vi "Numeric Limit Compare Runtime Test.vi"() -> (0 "error out":errorcluster, 2 "Pass":bool)   [LabVIEW 2015, in "Numeric Limit Compare Tests.lvlib"]
uses:
  Numeric Limit Compare Tests.lvlib
  Config/Comparison Types.ctl
  Config/Numeric Limit Compare Config.lvclass
  <vilib>/NI/Tag Bus/tag/Data Type.ctl
  <vilib>/NI/Tag Bus Module Framework/channel/channel classification.ctl
  classes/Step/Execution/StepState.ctl
  classes/Step/Execution/Step State Enum.ctl
  classes/Step/Execution/Step Flow Control.ctl
  Config/Numeric Limit Compare Config.lvclass/Numeric Limit Compare Config.ctl
  <vilib>/NI/Tag Bus/tag/tag descriptor.lvclass/tag descriptor.ctl
  <vilib>/NI/Tag Bus/table/data polymorphs/write one/write Double.vi
  <vilib>/NI/Tag Bus/table/data polymorphs/read one/read Boolean.vi
  Config/Write channel.vi
  Config/Write Comparison Type.vi
  Config/Write Lower Limit.vi
  Config/Write Negate Result.vi
  Config/Write Upper Limit_Limit.vi
  Config/Write Result Channel.vi
  <vilib>/NI/Tag Bus/tag/read tag name.vi
  <vilib>/NI/Tag Bus/tag/read data type.vi
  <vilib>/NI/Tag Bus/dictionary/locate tag.vi
  classes/Step/Execution/Step.lvclass
  <vilib>/NI/Tag Bus Module Framework/channel/TBM channel.lvclass
  <vilib>/NI/Tag Bus/tag/tag descriptor.lvclass
  <vilib>/NI/Tag Bus/dictionary/data dictionary.lvclass
  <vilib>/NI/Tag Bus/table/data table.lvlib
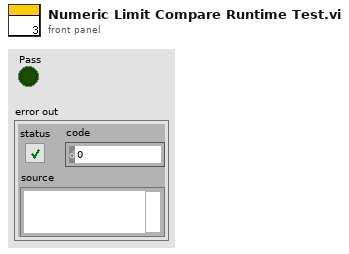
[diagram p1: front panel]
types:
  T1 = typedef "Comparison Types.ctl" = enum16{"GELE (>=<=)", "GTLE(><=)", "GTLT(><)", "GELT(>=<)", "EQ(==)", "NE (!=)", "GT(>)", "LT(<)", "GE(>=)", "LE(<=)"}
  T2 = typedef "Step.lvclass/StepState.ctl" = cluster{"Step State":T3, "Flow Control":T4, "Jump Index":i32}
  T3 = typedef "Step.lvclass/Step State Enum.ctl" = enum16{"Start", "Skipped", "Timeout", "Completed", "Running", "Aborted"}
  T4 = typedef "Step.lvclass/Step Flow Control.ctl" = enum16{"Next Step", "Jump"}
  T5 = typedef "TBM channel.lvclass/channel classification.ctl" = enum16{"input data", "output data", "processing parameter", "processing result"}
  T6 = typedef "tag bus.lvlib/tag descriptor.lvclass/Data Type.ctl" = enum16{"Double", "Single", "I64", "I32", "I16", "I8", "U64", "U32", "U16", "U8", "Boolean", "String", "Array of Double", "Array of Single", "Array of I64", "Array of I32", "Array of I16", "Array of I8", "Array of U64", "Array of U32", "Array of U16", "Array of U8", "Array of Boolean", "Array of String"}
  T7 = typedef "TBM channel.lvclass/data tables.ctl" = cluster{"input data":T8, "processing parameter":T8, "processing result":T8, "output data":T8}
  T8 = typedef "tag bus.lvlib/dictionary table pair.ctl" = cluster{"data dictionary":refnum<class "data dictionary.lvclass">, "data table":T9}
  T9 = typedef "tag bus.lvlib/data table.lvlib/data table.ctl" = cluster{"Double":dbl[], "Single":sgl[], "I64":i64[], "I32":i32[], "I16":i16[], "I8":i8[], "U64":u64[], "U32":u32[], "U16":u16[], "U8":u8[], "Boolean":bool[], "String":string[], "Array of Double":cluster{"DBL Array":dbl[]}[], "Array of Single":cluster{"SGL Array":sgl[]}[], "Array of I64":cluster{"I64 Array":i64[]}[], "Array of I32":cluster{"I32 Array":i32[]}[], "Array of I16":cluster{"I16 Array":i16[]}[], "Array of I8":cluster{"I8 Array":i8[]}[], "Array of U64":cluster{"U64 Array":u64[]}[], "Array of U32":cluster{"U32 Array":u32[]}[], "Array of U16":cluster{"U16 Array":u16[]}[], "Array of U8":cluster{"U8 Array":u8[]}[], "Array of Boolean":cluster{"Boolean Array":bool[]}[], "Array of String":cluster{"String Array":string[]}[]}
  T10 = cluster{"Step State":bool, "Flow Control":bool, "Jump Index":bool}
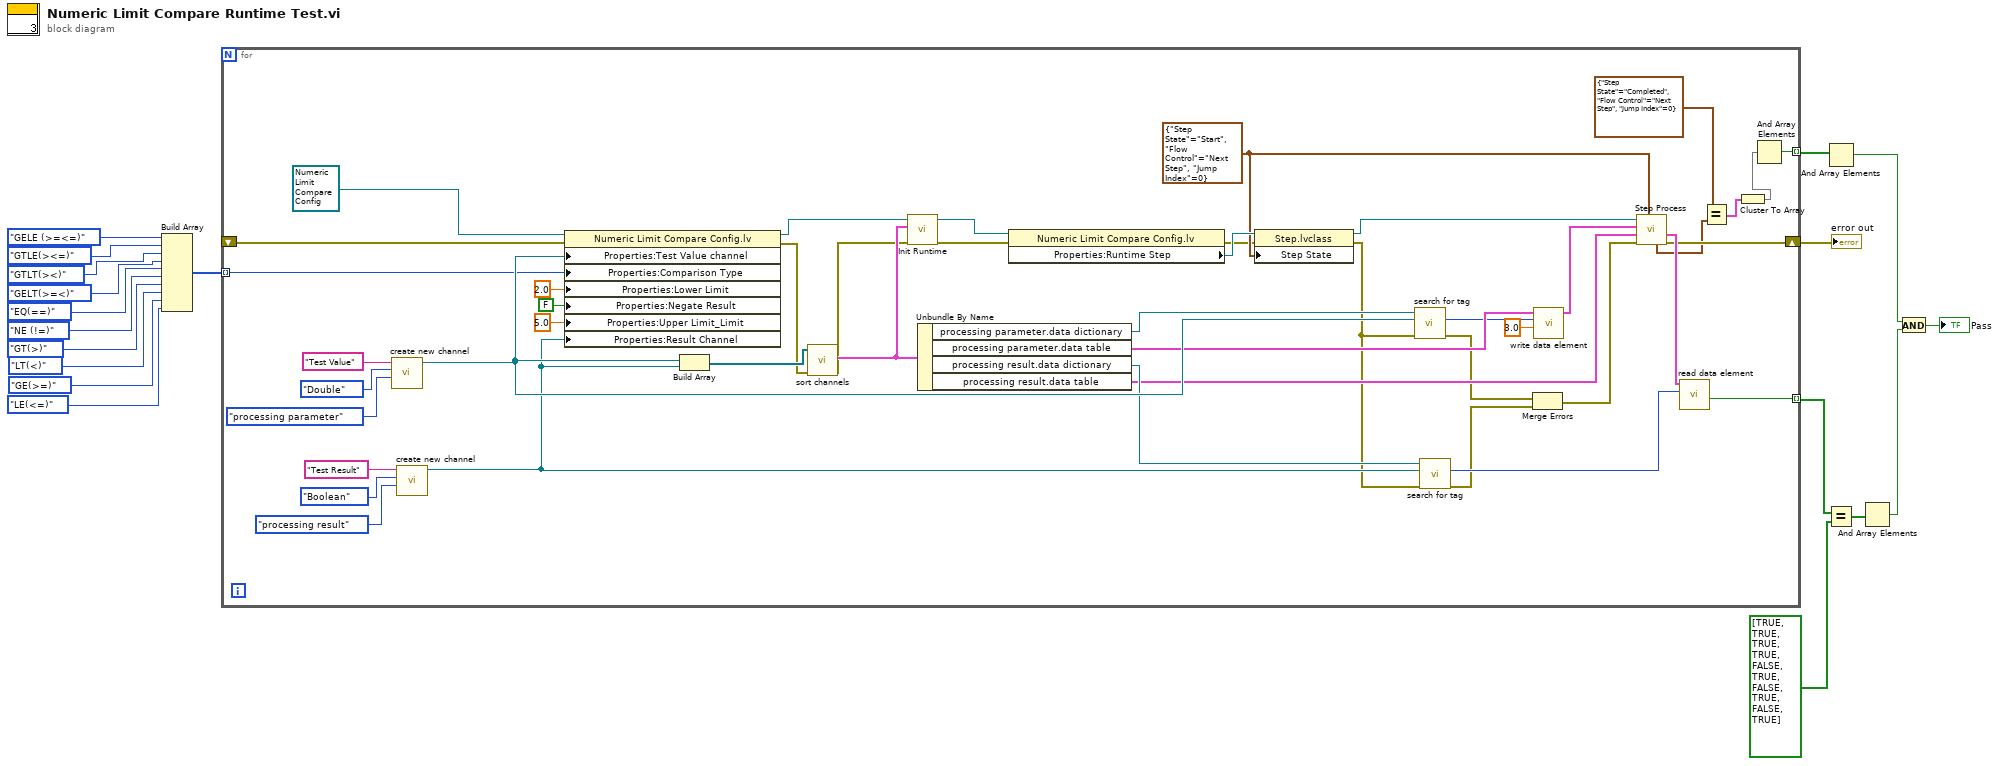
[diagram p0: block diagram]
diagram:
  n1 = Build Array(Comparison_Types."GELE (>=<=)" ("Comparison Type"), Comparison_Types."GTLE(><=)" ("Comparison Type"), Comparison_Types."GTLT(><)" ("Comparison Type"), Comparison_Types."GELT(>=<)" ("Comparison Type"), Comparison_Types."EQ(==)" ("Comparison Type"), Comparison_Types."NE (!=)" ("Comparison Type"), Comparison_Types."GT(>)" ("Comparison Type"), Comparison_Types."LT(<)" ("Comparison Type"), Comparison_Types."GE(>=)" ("Comparison Type"), Comparison_Types."LE(<=)" ("Comparison Type")) -> (w8:T1[])
  n2 = for {
    tunnel: [w28] -> w6 mode=indexing
    shift-right: [w33] -> w19
    shift-left: _ -> [w27]
    tunnel: w8 -> [w26] mode=indexing
    tunnel: [w20] -> w4 mode=indexing
    w55 = T2 {"Step State"=enum."Start", "Flow Control"=enum."Next Step", "Jump Index"=0} ("Step State")
    n3 = call <vilib>:"create new channel.vi"("channel classification"=channel_classification."processing parameter", "data type"=Data_Type."Double", "channel name"="Test Value") -> ("channel"=w53:refnum<class "TBM channel.lvclass">)  [unwired: 8 in]
    n4 = call <vilib>:"create new channel.vi"("channel classification"=channel_classification."processing result", "data type"=Data_Type."Boolean", "channel name"="Test Result") -> ("channel"=w43:refnum<class "TBM channel.lvclass">)  [unwired: 8 in]
    n5 = property class="Numeric Limit Compare Config.lv"(reference=refnum<class "Numeric Limit Compare Config.lvclass"> refnum ("Numeric Limit Compare Config.lvclass"), error in=w27, "Properties:Test Value channel"=w53, "Properties:Comparison Type"=w26, "Properties:Lower Limit"=2.0 ("Lower Limit"), "Properties:Negate Result"=FALSE ("Negate Result"), "Properties:Upper Limit_Limit"=5.0 ("Upper Limit_Limit"), "Properties:Result Channel"=w43) -> (reference out=w63:refnum<class "Numeric Limit Compare Config.lvclass">, error out=w37:errorcluster)
    n6 = Build Array(w53, w43) -> (w59:refnum<class "TBM channel.lvclass">[])
    n7 = call <vilib>:"sort channels.vi"("error in"=w37, "channels in"=w59) -> ("error out"=w36:errorcluster, "data allocations"=w40:T7)  [unwired: 7 in, 1 out]
    n8 = call-dynamic "Init Runtime.vi"("error in (no error)"=w36, "data allocations"=w40, "Numeric Limit Compare Config in"=w63) -> ("error out"=w35:errorcluster, "Numeric Limit Compare Config out"=w58:refnum<class "Numeric Limit Compare Config.lvclass">)  [unwired: 6 in, 1 out]
    n9 = Unbundle By Name(w40) -> ("processing parameter.data dictionary"=w54:refnum<class "data dictionary.lvclass">, "processing parameter.data table"=w52:T9, "processing result.data dictionary"=w44:refnum<class "data dictionary.lvclass">, "processing result.data table"=w42:T9)
    n10 = property class="Numeric Limit Compare Config.lv"(reference=w58, error in=w35) -> (error out=w34:errorcluster, "Properties:Runtime Step"=w57:refnum<class "Step.lvclass">)  [unwired: 1 out]
    n11 = property class="Step.lvclass"(reference=w57, error in=w34, "Step State"=w55) -> (reference out=w56:refnum<class "Step.lvclass">, error out=w32:errorcluster)
    n12 = call <vilib>:"search for tag.vi"("error in"=w32, "system tag"=w53, "data dictionary in"=w54) -> ("error out"=w30:errorcluster, "index"=w51:i32)  [unwired: 6 in, 1 out]
    n13 = call <vilib>:"search for tag.vi"("error in"=w32, "system tag"=w43, "data dictionary in"=w44) -> ("error out"=w31:errorcluster, "index"=w41:i32)  [unwired: 6 in, 1 out]
    n14 = Merge Errors(w30, w31) -> (w29:errorcluster)
    n15 = call-poly <vilib>:"write data element.vi"("value"=3.0, "index"=w51, "data table in"=w52) -> ("data table out"=w39:T9)  [unwired: 8 in]
    n16 = call-dynamic "Step Process.vi"("Step State in"=w55, "error in (no error)"=w29, "result allocation"=w42, "parameters"=w39, "Step in"=w56) -> ("error out"=w33:errorcluster, "results"=w38:T9, "Step State out"=w24:T2)  [unwired: 2 in, 2 out]
    n17 = call-poly <vilib>:"read data element.vi"("index"=w41, "data table in"=w38) -> ("value"=w28:bool)  [unwired: 8 in, 1 out]
    n18 = Equal?(x=T2 {"Step State"=enum."Completed", "Flow Control"=enum."Next Step", "Jump Index"=0}, y=w24) -> (x = y?=w22:T10)
    n19 = Cluster To Array(cluster=w22) -> (array=w21:bool[])
    n20 = And Array Elements(Boolean array=w21) -> (logical AND=w20:bool)
  }
  "error out" <- w19
  n21 = And Array Elements(Boolean array=w4) -> (logical AND=w2:bool)
  n22 = Equal?(x=w6, y=bool[] [TRUE, TRUE, TRUE, TRUE, FALSE, TRUE, FALSE, TRUE, FALSE, TRUE]) -> (x = y?=w5:bool[])
  n23 = And Array Elements(Boolean array=w5) -> (logical AND=w3:bool)
  n24 = And(x=w2, y=w3) -> (x .and. y?=→"Pass":bool)
